vi "sensor cmd use calibration.vi"(10 "useCalibration":bool, 11 "device_handle":u32) -> (2 "function return":i32, 3 "device_handle out":u32)   [LabVIEW 2019, in "apdm.lvlib"]
doc: "APDM_EXPORT int apdm_sensor_cmd_use_calibration(apdm_device_handle_t device_handle, bool useCalibration);"
uses:
  apdm.lvlib
  Lee Lab/CP FES Walking 2018/Code/Working/LabVIEW/apdm.dll
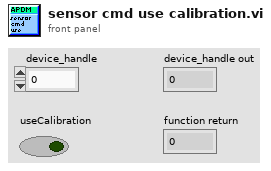
[diagram p1: front panel]
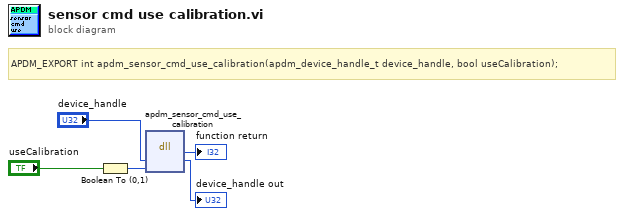
[diagram p0: block diagram]
diagram:
  # "APDM_EXPORT int apdm_sensor_cmd_use_calibration(apdm_device_handle_t device_handle, bool useCalibration);"
  n1 = Boolean To (0,1)(Boolean="useCalibration") -> (0, 1=w1:i16)
  n2 = dll-call lib="C:/Users/jfalesi/Dropbox/Lee Lab/CP FES Walking 2018/Code/Working/LabVIEW/apdm.*" fn="apdm_sensor_cmd_use_calibration"("device_handle"="device_handle", "useCalibration"=w1) -> (→"function return":i32, "device_handle"=→"device_handle out":u32)  [unwired: 4 in, 2 out]
